vi "Convert FP to Hex.vi"(11 "Number":sgl=-101.101 format="%.12f") -> (3 "hex integer string":string)   [LabVIEW 2018, in "Meerstetter Lib.lvlib" / "Meerstetter TEC.lvclass"]
doc: "This VI shows how LabVIEW stores SGL floating-point numbers in memory in binary format. The 32-bit binary number is based on the following IEEE 754 format:\n\n1 bit for the SIGN\n8 bits for the EXPONENT\n23 bits for the MANTISSA\n\nThe formula for the conversion is the following:\n\nSGL = (-1)^SIGN * 1.MANTISSA * 2^(EXPONENT-127)\n\nYou can use this VI to convert SGL numbers to their binary storage equivalent, and vice versa."
uses:
  Meerstetter TEC.lvclass
panel:
  out "Sign":bool=TRUE
  out "Mantissa":bool[](array[boolean])=[TRUE, FALSE, FALSE, TRUE, FALSE, TRUE, FALSE, FALSE, FALSE, TRUE, TRUE, FALSE, FALSE, TRUE, TRUE, TRUE, FALSE, TRUE, TRUE, FALSE, TRUE, TRUE, FALSE]
  out "Exponent":bool[](array[boolean])=[TRUE, FALSE, FALSE, FALSE, FALSE, TRUE, FALSE, TRUE]
  out "Exponent":sgl=6.0 format="%.2f"
  out "Mantissa":sgl=1.5797031 format="%.8f"
  # "SGL to Binary Storage Format"
  # "Enter Decimal Number -->"
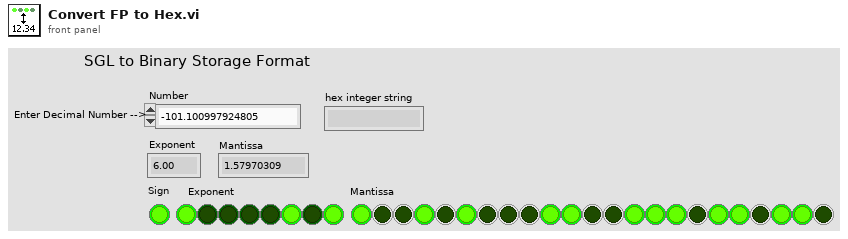
[diagram p1: front panel]
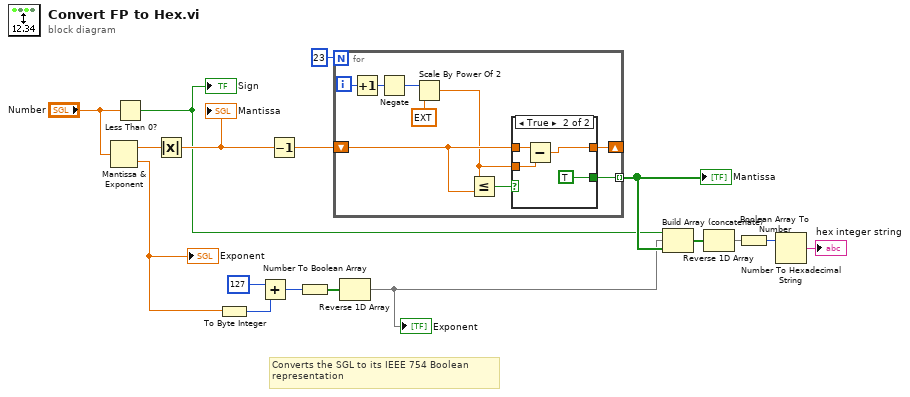
[diagram p0: block diagram]
diagram:
  # "Converts the SGL to its IEEE 754 Boolean \nrepresentation"
  n1 = Mantissa & Exponent(0:"Number") -> (1:w8:sgl, 2:w11:sgl)
  "Exponent" <- w11
  n2 = Less Than 0?(x="Number") -> (x < 0?=w5:bool)
  "Sign" <- w5
  n3 = Absolute Value(x=w8) -> (abs(x)=w9:sgl)
  "Mantissa" <- w9
  n4 = To Byte Integer(number=w11) -> (8bit integer=w17:i8)
  n5 = Add(x=i8 127, y=w17) -> (x+y=w16:i8)
  n6 = Decrement(x=w9) -> (x-1=w13:sgl)
  n7 = Number To Boolean Array(number=w16) -> (Boolean array=w15:bool[])
  n8 = for {
    N: 23 -> [_]
    shift-right: [w19] -> _
    shift-left: w13 -> [w21]
    tunnel: [w18] -> w7 mode=indexing
    i -> [w26]
    n9 = Increment(x=w26) -> (x+1=w25:i32)
    n10 = Negate(x=w25) -> (-x=w24:i32)
    n11 = Scale By Power Of 2(n=w24, x=ext 1.0) -> (x*2^n=w20:ext)
    n12 = Less Or Equal?(x=w20, y=w21) -> (x <= y?=w22:bool)
    n13 = case shown="True" w22 {
      tunnel: w21 -> [w27 w32]
      tunnel: w20 -> [_ w29]
      tunnel: [w27 w31] -> w19
      tunnel: [FALSE TRUE] -> w18
      frame False {
      }
      frame True {
        n14 = Subtract(x=w32, y=w29) -> (x-y=w31:ext)
      }
    }
  }
  "Mantissa" <- w7
  n15 = Reverse 1D Array(array=w15) -> (reversed array=w6:bool[])
  "Exponent" <- w6
  n16 = Build Array (concatenate)(w5, w6, w7) -> (w2:bool[])
  n17 = Reverse 1D Array(array=w2) -> (reversed array=w1:bool[])
  n18 = Boolean Array To Number(Boolean array=w1) -> (number=w4:u32)
  n19 = Number To Hexadecimal String(2:w4) -> (0:→"hex integer string":string)  [unwired: 1 in]
